vi "Get XML Tag.vi"(8 "error in (no error)":errorcluster, 9 "Ignore XML Comments (T)":bool=TRUE, 10 "Tag name":string, 11 "XML String in":string) -> (0 "error out":errorcluster, 1 "Remaining string":string, 2 "Tag value":string, 3 "XML String dup":string, 5 "Tag attributes":string)   [LabVIEW 2015, in "NI_Azure_XML Parsing.lvlib"]
uses:
  NI_Azure_XML Parsing.lvlib
  <vilib>/regexp/Match Regular Expression.xnode
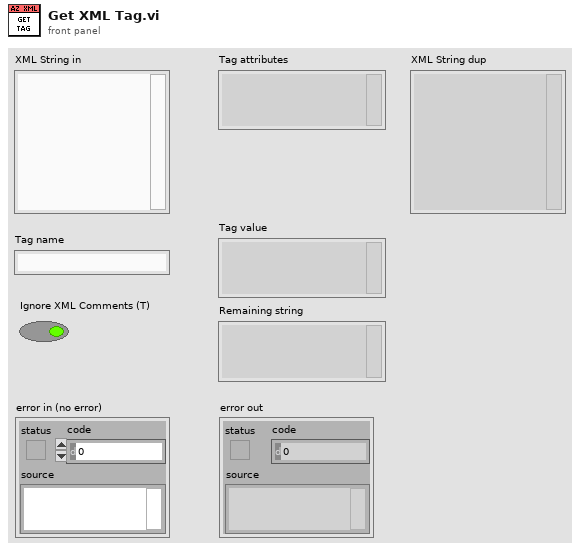
[diagram p1: front panel]
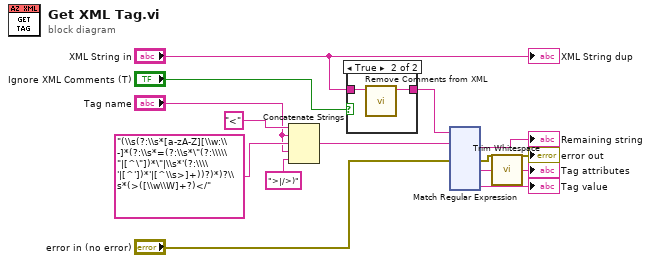
[diagram p0: block diagram]
diagram:
  n1 = Concatenate Strings("<", "Tag name", "(\\s(?:\\s*[a-zA-Z][\\w:\\-]*(?:\\s*=(?:\\s*\"(?:\\\\\"|[^\"])*\"|\\s*'(?:\\\\'|[^'])*'|[^\\s>]+))?)*)?\\s*(>([\\w\\W]+?)</", "Tag name", ">|/>)" ("string")) -> (w10:string)
  n2 = case shown="True" "Ignore XML Comments (T)" {
    tunnel: "XML String in" -> [w15 w17]
    tunnel: [w15 w16] -> w1
    frame False {
    }
    frame True {
      n3 = call "Remove Comments from XML.vi"("XML String in"=w17) -> ("XML String out"=w16:string)  [unwired: 10 in]
    }
  }
  n4 = xnode "Match Regular Expression"("input string"=w1, "regular expression"=w10, "error in"="error in (no error)") -> ("after match"=→"Remaining string":string, "error out"=→"error out":errorcluster, "submatch 1"=w5:string, "submatch 3"=→"Tag value":string)  [unwired: 3 in, 4 out]
  n5 = call <vilib>:"Trim Whitespace.vi"("string"=w5) -> ("trimmed string"=→"Tag attributes":string)  [unwired: 1 in]
  "XML String dup" <- "XML String in"
